vi "focus checker_file.vi"() -> ()   [LabVIEW 2020]
uses:
  <vilib>/vision/Management.llb/Cast Image 2 Method.ctl
  <vilib>/vision/NI_Vision_Development_Module.lvlib
panel:
  out "Circles (Shape Detection 1) 2":T1(array[cluster]) {"Position"."Y" format="%.2f"; "Position"."X" format="%.2f"}
  out "Filtered Image 4":T2(plugin-control)
  out "Circles (Shape Detection 1)":T1(array[cluster]) {"Position"."Y" format="%.2f"; "Position"."X" format="%.2f"}
  out "Filtered Image 3":T2(plugin-control)
  out "Filtered Image 2":T2(plugin-control)
  in  "Filter Parameters":T3={"Sigma"=1.0, "HThresh"=0.7, "LThres"=0.2, "WindowSize"=9} {"LThres" min=0 max=1 format="%.2f"; "HThresh" min=0 max=1 format="%.2f"; "Sigma" min=0 max=1 format="%.2f"}
  out "Annulus 2":T4 {"End Angle" min=-90.0 max=90.0 step=1.0 format="%.2f"; "Start Angle" min=-90.0 max=90.0 step=1.0 format="%.2f"; "Center X" scale=0.0..1024.0}
  out "Particle Measurements (Pixels)":dbl[][](array[numeric]) format="%.2f"
  out "Histogram":T5(graph)
  out "Number of Particles":i32
  out "Binary Image":T2(plugin-control)
  in  "LUT1":cluster{u16, u16}(slide)={0, 4095} caption="Slide" scale=0.0..4095.0
  in  "File Path":path
  in  "Filter Type":T6(ring)
  out "Mean Value":sgl format="%.2f"
  out "Filtered Image":T2(plugin-control)
  out "Acquired Image":T2(plugin-control)
  in  "stop":bool
  # "The larger this value, the sharper the image.  The sharper the image,\nthe more in focus the camera is."
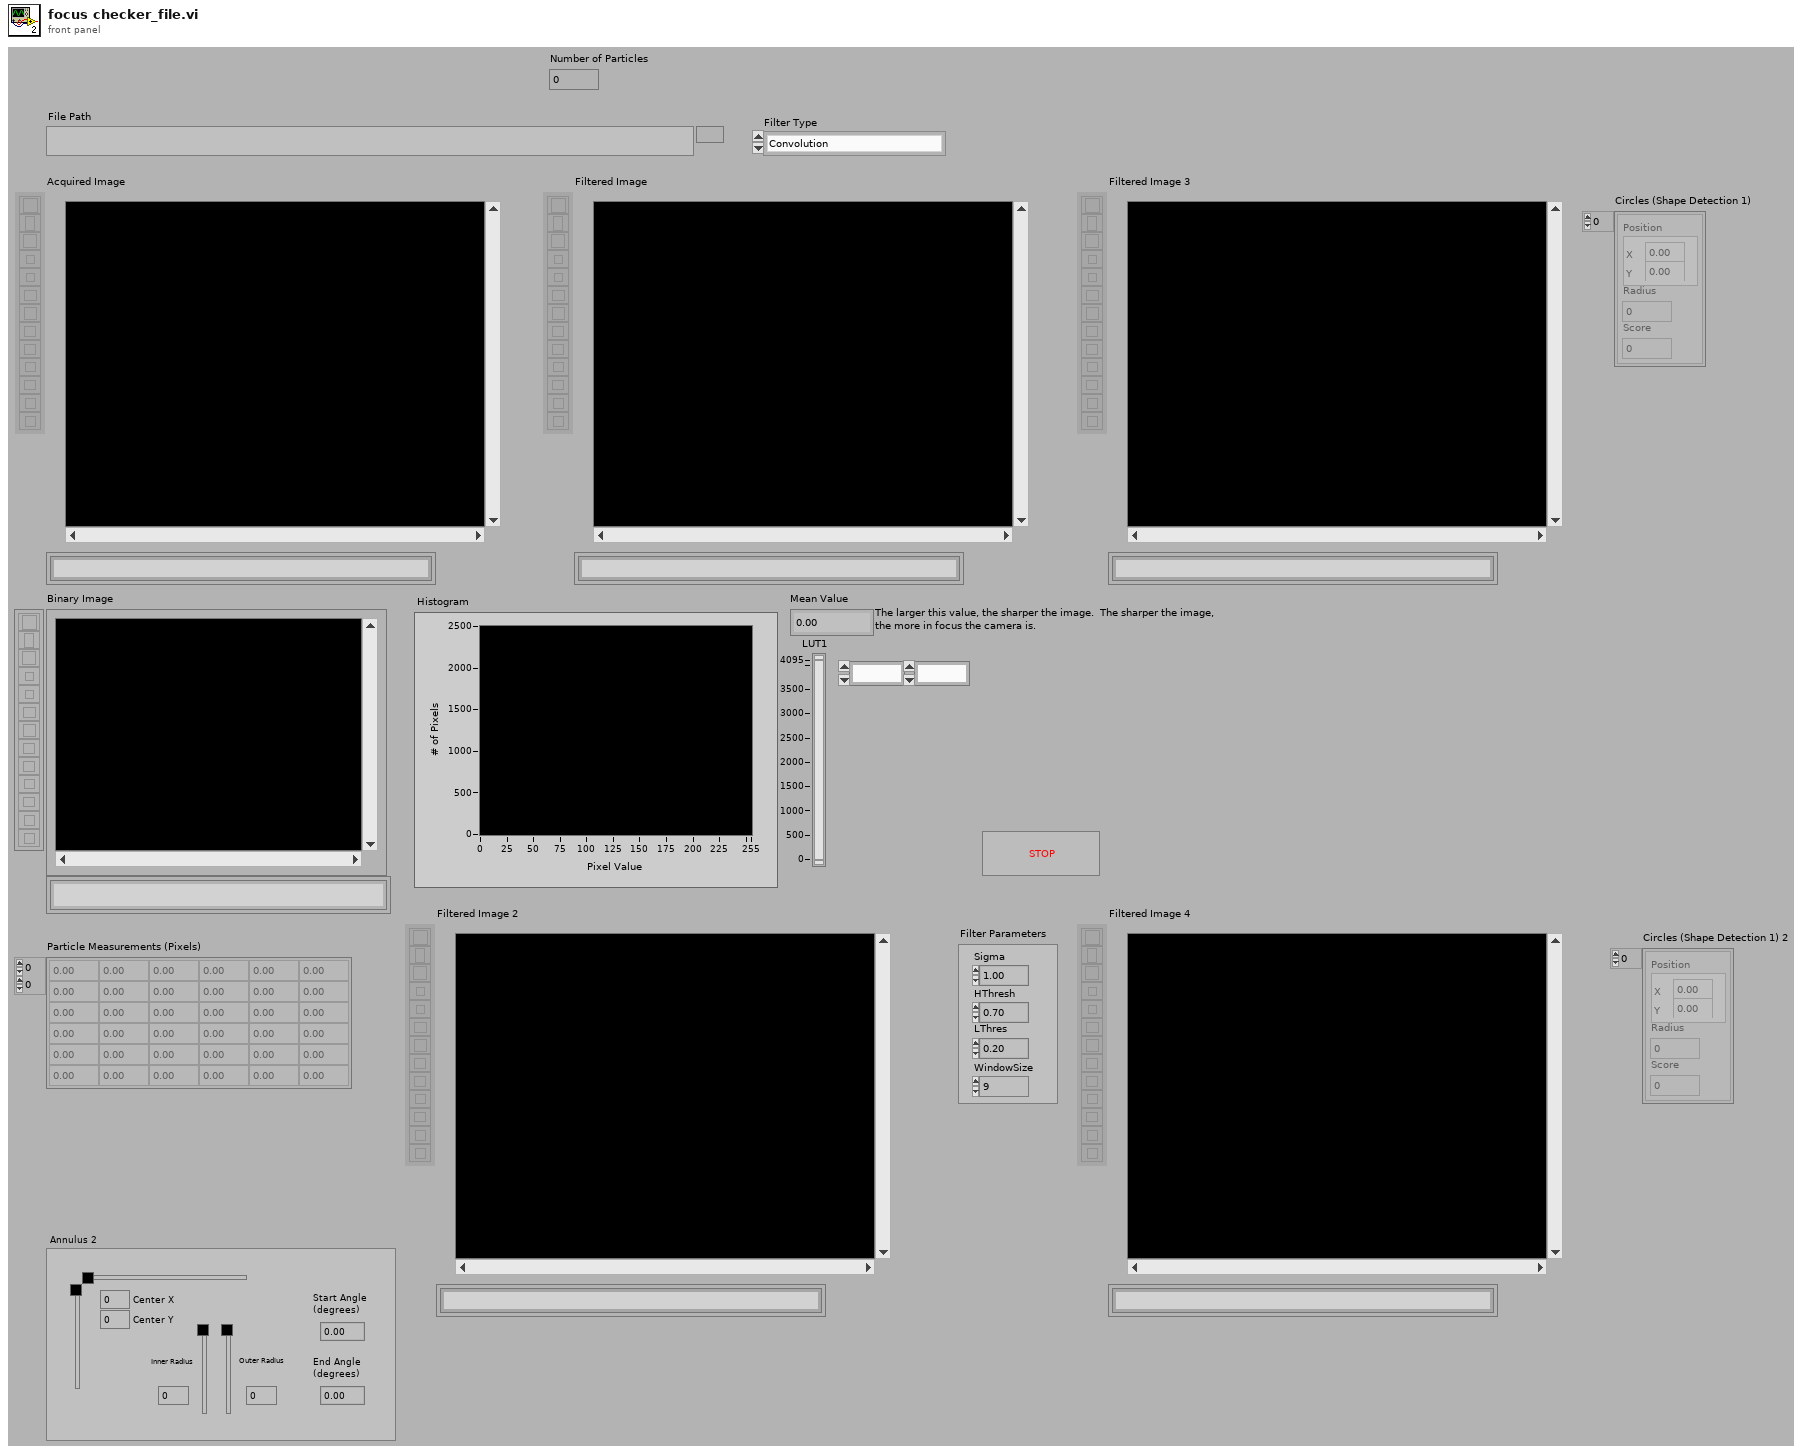
[diagram p1: front panel]
types:
  T1 = cluster{"Position":cluster{"X":sgl, "Y":sgl}, "Radius":dbl, "Score":dbl}[]
  T2 = typedef "IMAQ Image.ctl" = refnum<image>
  T3 = cluster{"Sigma":sgl, "HThresh":sgl, "LThres":sgl, "WindowSize":i32}
  T4 = typedef "IMAQ Circle" = cluster{"Center X":i32, "Center Y":i32, "Inner Radius":i32, "Outer Radius":i32, "Start Angle":dbl, "End Angle":dbl}
  T5 = cluster{"Starting Value":sgl, "Incremental Value":sgl, "Histogram":u32[]}
  T6 = enum16{"Convolution", "Differentiation", "Gradient", "Prewitt", "Roberts", "Sigma", "Sobel"}
  T7 = typedef "Image Type" = u32
  T8 = enum32{"Differentiation", "Gradient", "Prewitt", "Roberts", "Sigma", "Sobel"}
  T9 = typedef "Cast Image 2 Method.ctl" = u32
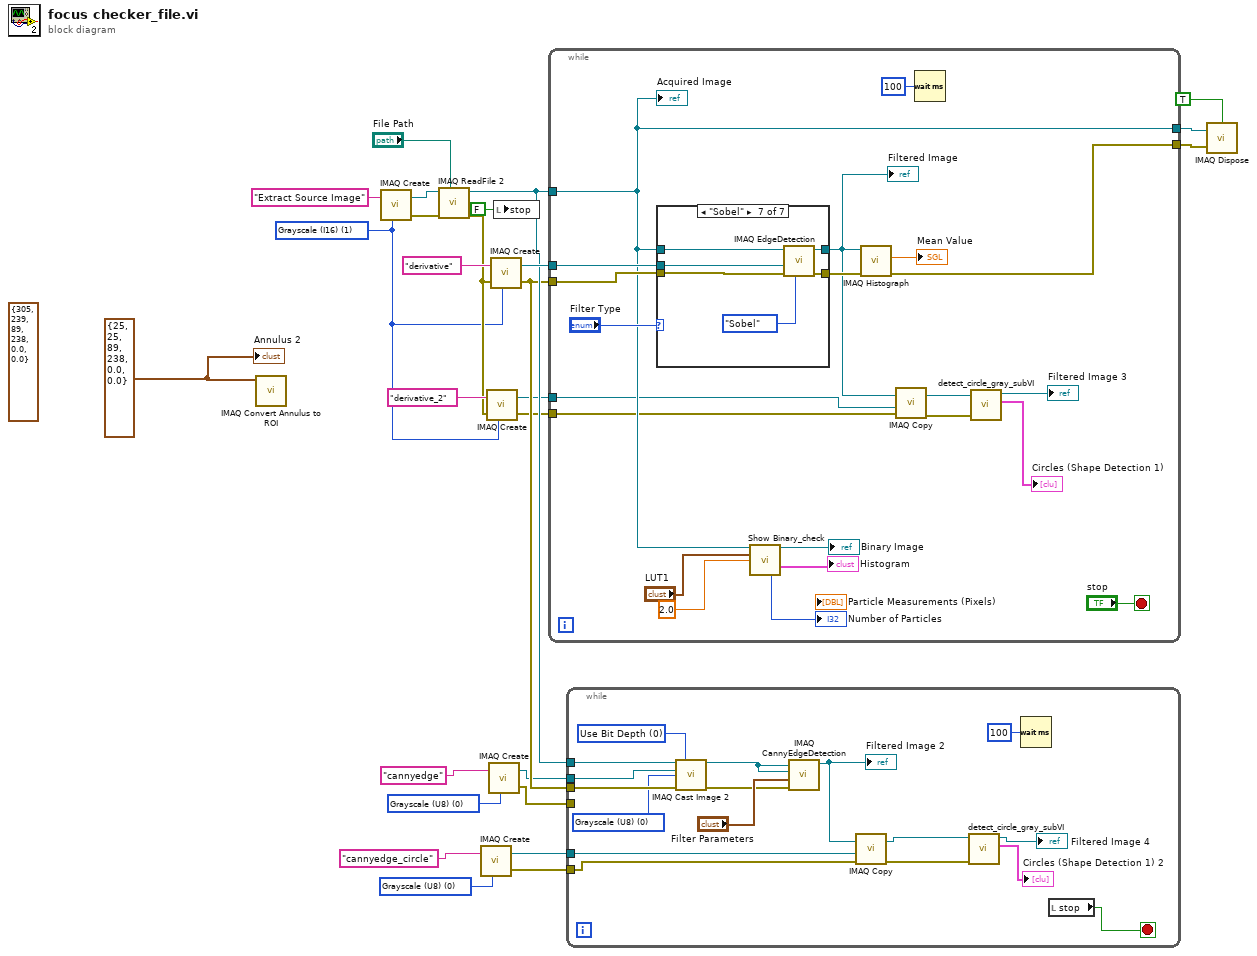
[diagram p0: block diagram]
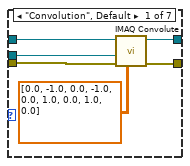
[diagram p2: hidden frame]
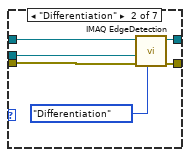
[diagram p3: hidden frame]
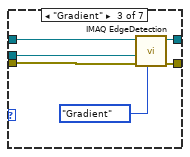
[diagram p4: hidden frame]
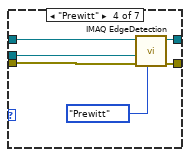
[diagram p5: hidden frame]
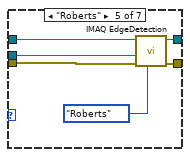
[diagram p6: hidden frame]
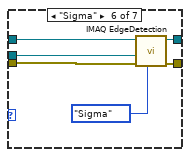
[diagram p7: hidden frame]
diagram:
  w4 = T7 0 items=["Grayscale (U8)", "Grayscale (I16)", "Grayscale (SGL)", "Complex (CSG)", "RGB (U32)", "HSL (U32)", "RGB (U64)", "Grayscale (U16)"] ("Image Type")
  w13 = T7 0 items=["Grayscale (U8)", "Grayscale (I16)", "Grayscale (SGL)", "Complex (CSG)", "RGB (U32)", "HSL (U32)", "RGB (U64)", "Grayscale (U16)"] ("Image Type")
  (unwired) T4 {"Center X"=305, "Center Y"=239, "Inner Radius"=89, "Outer Radius"=238, "Start Angle"=0.0, "End Angle"=0.0} ("Annulus")
  w17 = T4 {"Center X"=25, "Center Y"=25, "Inner Radius"=89, "Outer Radius"=238, "Start Angle"=0.0, "End Angle"=0.0} ("Annulus")
  w7 = T7 1 items=["Grayscale (U8)", "Grayscale (I16)", "Grayscale (SGL)", "Complex (CSG)", "RGB (U32)", "HSL (U32)", "RGB (U64)", "Grayscale (U16)"] ("Image Type")
  n1 = call "IMAQ Convert Annulus to ROI"("Annulus"=w17) -> ()  [unwired: 8 in, 2 out]
  n2 = call "IMAQ Create"("Image Name"="Extract Source Image", "Image Type"=w7) -> ("New Image"=w22:T2, "error out"=w21:errorcluster)  [unwired: 3 in]
  n3 = call "IMAQ ReadFile 2"("File Path"="File Path", "error in (no error)"=w21, "Image"=w22) -> ("error out"=w8:errorcluster, "Image Out"=w16:T2)  [unwired: 4 in, 3 out]
  n4 = call "IMAQ Create"("Image Name"="cannyedge_circle", "Image Type"=w4) -> ("New Image"=w2:T2, "error out"=w1:errorcluster)  [unwired: 3 in]
  n5 = call "IMAQ Create"("Image Name"="derivative_2", "Image Type"=w7, "error in (no error)"=w8) -> ("New Image"=w6:T2, "error out"=w5:errorcluster)  [unwired: 2 in]
  n6 = call "IMAQ Create"("Image Name"="cannyedge", "Image Type"=w13) -> ("New Image"=w12:T2, "error out"=w11:errorcluster)  [unwired: 3 in]
  n7 = call "IMAQ Create"("Image Name"="derivative", "Image Type"=w7, "error in (no error)"=w8) -> ("New Image"=w25:T2, "error out"=w15:errorcluster)  [unwired: 2 in]
  n8 = local write "stop"(FALSE ("stop")) -> ()
  n9 = while {
    tunnel: w16 -> [w38]
    tunnel: [w42] -> w19
    tunnel: w25 -> [w45]
    tunnel: w15 -> [w40]
    tunnel: [w38] -> w18
    tunnel: w6 -> [w32]
    tunnel: w5 -> [w33]
    stop <- "stop" stop-if-true
    n10 = case shown="\"Sobel\"" "Filter Type" {
      tunnel: w38 -> [w52 w58 w64 w70 w76 w82 w88]
      tunnel: w40 -> [w51 w57 w63 w69 w75 w81 w87]
      tunnel: w45 -> [w50 w59 w65 w71 w77 w83 w89]
      tunnel: [w49 w54 w60 w66 w72 w78 w84] -> w44
      tunnel: [w48 w55 w61 w67 w73 w79 w85] -> w31
      frame "Convolution", Default {
        n11 = call "IMAQ Convolute"("Kernel"=sgl[][] [[0.0, -1.0, 0.0], [-1.0, 0.0, 1.0], [0.0, 1.0, 0.0]], "error in (no error)"=w51, "Image Dst"=w50, "Image Src"=w52) -> ("error out"=w49:errorcluster, "Image Dst Out"=w48:T2)  [unwired: 6 in]
      }
      frame "Differentiation" {
        n12 = call "IMAQ EdgeDetection"("Method"=T8."Differentiation", "error in (no error)"=w57, "Image Dst"=w59, "Image Src"=w58) -> ("error out"=w54:errorcluster, "Image Dst Out"=w55:T2)  [unwired: 6 in]
      }
      frame "Gradient" {
        n13 = call "IMAQ EdgeDetection"("Method"=T8."Gradient", "error in (no error)"=w63, "Image Dst"=w65, "Image Src"=w64) -> ("error out"=w60:errorcluster, "Image Dst Out"=w61:T2)  [unwired: 6 in]
      }
      frame "Prewitt" {
        n14 = call "IMAQ EdgeDetection"("Method"=T8."Prewitt", "error in (no error)"=w69, "Image Dst"=w71, "Image Src"=w70) -> ("error out"=w66:errorcluster, "Image Dst Out"=w67:T2)  [unwired: 6 in]
      }
      frame "Roberts" {
        n15 = call "IMAQ EdgeDetection"("Method"=T8."Roberts", "error in (no error)"=w75, "Image Dst"=w77, "Image Src"=w76) -> ("error out"=w72:errorcluster, "Image Dst Out"=w73:T2)  [unwired: 6 in]
      }
      frame "Sigma" {
        n16 = call "IMAQ EdgeDetection"("Method"=T8."Sigma", "error in (no error)"=w81, "Image Dst"=w83, "Image Src"=w82) -> ("error out"=w78:errorcluster, "Image Dst Out"=w79:T2)  [unwired: 6 in]
      }
      frame "Sobel" {
        n17 = call "IMAQ EdgeDetection"("Method"=T8."Sobel", "error in (no error)"=w87, "Image Dst"=w89, "Image Src"=w88) -> ("error out"=w84:errorcluster, "Image Dst Out"=w85:T2)  [unwired: 6 in]
      }
    }
    "Filtered Image" <- w31
    n18 = call "Show Binary_check.vi"("Input Image"=w38, "LUT1"="LUT1", "Boundary"=2.0) -> ("Binary Image"=→"Binary Image":T2, "Histogram Graph"=→"Histogram":T5, "Number of Particles"=→"Number of Particles":i32)  [unwired: 8 in, 2 out]
    n19 = call "IMAQ Histograph"("error in (no error)"=w44, "Image"=w31) -> ("error out"=w42:errorcluster, "Mean Value"=→"Mean Value":sgl)  [unwired: 6 in, 2 out]
    n20 = call "IMAQ Copy"("error in (no error)"=w33, "Image Dst"=w32, "Image Src"=w31) -> ("error out"=w29:errorcluster, "Image Dst Out"=w30:T2)  [unwired: 3 in]
    n21 = Wait (ms)(milliseconds to wait=u32 100) -> ()  [unwired: 1 out]
    n22 = call "detect_circle_gray_subVI.vi"("error in (no error)"=w29, "Image Out 2"=w30) -> ("Circles (Shape Detection 1)"=→"Circles (Shape Detection 1)":T1, "Image Out"=→"Filtered Image 3":T2)  [unwired: 7 in, 1 out]
    "Acquired Image" <- w38
  }
  n23 = while {
    tunnel: w16 -> [w102]
    tunnel: w15 -> [w103]
    tunnel: w12 -> [w97]
    tunnel: w11 -> [_]
    tunnel: w2 -> [w95]
    tunnel: w1 -> [w94]
    stop <- w104 stop-if-true
    w100 = T9 0 items=["Use Bit Depth", "Shift", "Use Lookup Table"] ("Method")
    w101 = T7 0 items=["Grayscale (U8)", "Grayscale (I16)", "Grayscale (SGL)", "Complex (CSG)", "RGB (U32)", "HSL (U32)", "RGB (U64)", "Grayscale (U16)"] ("Image Type")
    n24 = call "IMAQ Cast Image 2"("Image Src"=w102, "Method"=w100, "Image Dst"=w97, "Image Type"=w101, "error in (no error)"=w103) -> ("Image Dst Out"=w99:T2, "error out"=w98:errorcluster)  [unwired: 9 in]
    n25 = call "IMAQ CannyEdgeDetection"("Image Src"=w99, "Image Dst"=w99, "Filter Parameters"="Filter Parameters", "error in (no error)"=w98) -> ("Image Dst Out"=w96:T2)  [unwired: 4 in, 1 out]
    "Filtered Image 2" <- w96
    n26 = call "IMAQ Copy"("error in (no error)"=w94, "Image Dst"=w95, "Image Src"=w96) -> ("error out"=w92:errorcluster, "Image Dst Out"=w93:T2)  [unwired: 3 in]
    n27 = call "detect_circle_gray_subVI.vi"("error in (no error)"=w92, "Image Out 2"=w93) -> ("Circles (Shape Detection 1)"=→"Circles (Shape Detection 1) 2":T1, "Image Out"=→"Filtered Image 4":T2)  [unwired: 7 in, 1 out]
    n28 = Wait (ms)(milliseconds to wait=u32 100) -> ()  [unwired: 1 out]
    n29 = local read "stop"() -> (w104:bool)
  }
  n30 = call "IMAQ Dispose"("All Images? (No)"=TRUE, "Image"=w18, "error in (no error)"=w19) -> ()  [unwired: 3 in, 1 out]
  "Annulus 2" <- w17
